vi "CH_LM Config Position Stability Cycle Duration.vi"(0 "Meter Index":i32, 2 "Cycle Time (00:01:00)":T1={"Hours"=0, "Minutes"=1, "Seconds"=0}, 5 "error in (no error)":errorcluster, 7 "Timeout / ms (3000)":i32=3000, 8 "Action (query)":bool, 9 "Lock Timeout / ms (1000)":i32=1000) -> (11 "Lock timed out":bool, 14 "Meter Index":i32, 16 "Cycle Time":T1={"Hours"=0, "Minutes"=1, "Seconds"=0}, 19 "error out":errorcluster)   [LabVIEW 2012, in "CH_LM.lvlib"]
doc: "This command will set/query the position stability cycle time, which takes effect at the end of the current position stability cycle.\n\n<B>Attention:</B> This command will apply only when a quadrant thermopile probe is attached in one of the position stability display modes."
uses:
  CH_LM.lvlib
  CH_LM Time.ctl
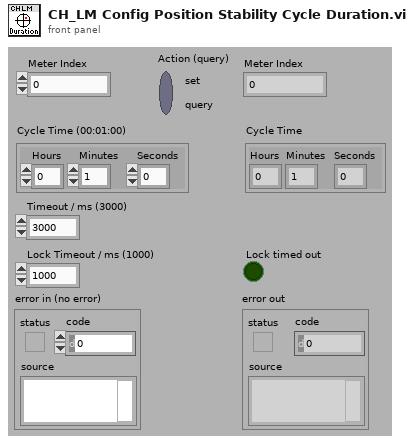
[diagram p1: front panel]
types:
  T1 = typedef "CH_LM.lvlib/CH_LM Time.ctl" = cluster{"Hours":i32, "Minutes":i32, "Seconds":i32}
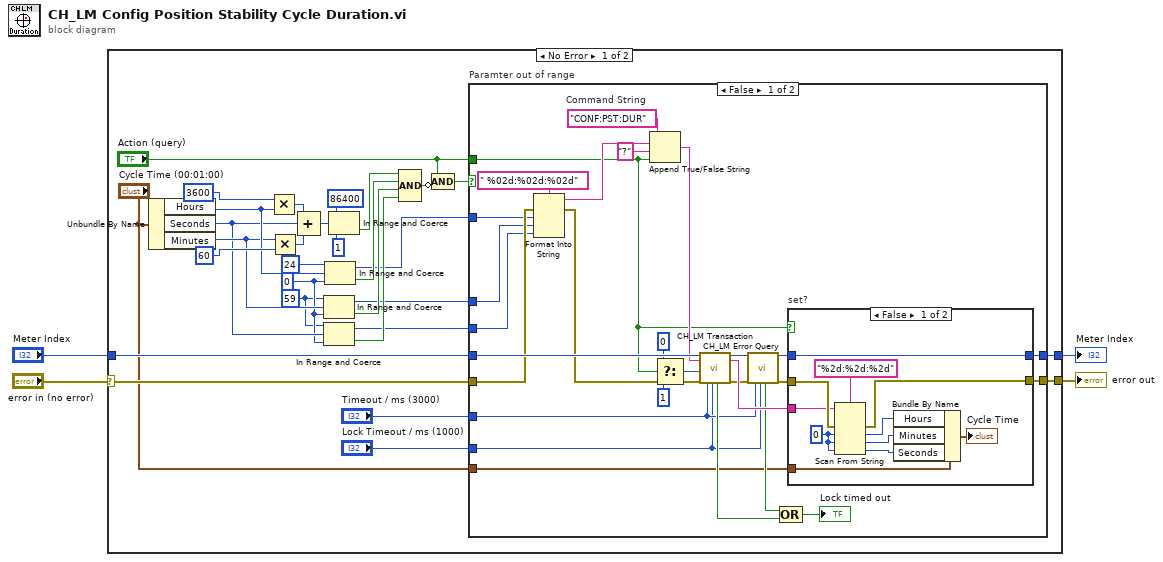
[diagram p0: block diagram]
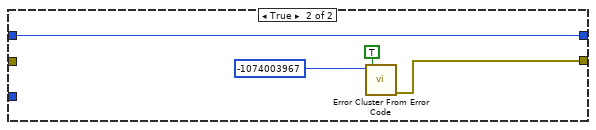
[diagram p3: hidden frame]
diagram:
  n1 = case shown="No Error" "error in (no error)" {
    selector: "error in (no error)" -> [w34 w81]
    tunnel: [w32 w81] -> w4
    tunnel: "Meter Index" -> [w33 w80]
    tunnel: [w31 w80] -> w1
    frame No Error {
      w13 = 59 ("upper limit")
      w14 = 0 ("lower limit")
      n2 = Unbundle By Name("Cycle Time (00:01:00)") -> ("Hours"=w17:i32, "Seconds"=w15:i32, "Minutes"=w16:i32)
      n3 = Multiply(x=3600, y=w17) -> (x*y=w23:i32)
      n4 = Multiply(x=w16, y=60) -> (x*y=w22:i32)
      n5 = Compound Arithmetic op=ADD(w23, w15, w22) -> (w21:i32)
      n6 = In Range and Coerce(upper limit=w13, x=w16, lower limit=w14) -> (coerced(x)=w6:i32, In Range?=w9:bool)
      n7 = In Range and Coerce(upper limit=w13, x=w15, lower limit=w14) -> (coerced(x)=w5:i32, In Range?=w8:bool)
      n8 = In Range and Coerce(upper limit=24, x=w17, lower limit=w14) -> (coerced(x)=w7:i32, In Range?=w10:bool)
      n9 = In Range and Coerce(upper limit=86400, x=w21, lower limit=1) -> (In Range?=w11:bool)  [unwired: 1 out]
      n10 = Compound Arithmetic op=AND(w11, w10, w9, w8) -> (w12:bool)
      n11 = Compound Arithmetic op=AND("Action (query)", invert w12) -> (w26:bool)
      n12 = case "Paramter out of range" shown="False" w26 {
        tunnel: w34 -> [w50 _]
        tunnel: w33 -> [w62 w79]
        tunnel: [w59 w77] -> w32
        tunnel: [w56 w79] -> w31
        tunnel: "Timeout / ms (3000)" -> [w42 _]
        tunnel: "Lock Timeout / ms (1000)" -> [w41 _]
        tunnel: w7 -> [w47 _]
        tunnel: "Action (query)" -> [w39 _]
        tunnel: "Cycle Time (00:01:00)" -> [w43 _]
        tunnel: w6 -> [w45 _]
        tunnel: w5 -> [w44 _]
        frame False {
          w61 = "CONF:PST:DUR"  # Command String
          n13 = Format Into String(format string=" %02d:%02d:%02d", error in=w50, w47, w45, w44) -> (resulting string=w48:string, error out=w37:errorcluster)  [unwired: 1 in]
          n14 = Append True/False String(1:w39, 2:"?" ("true string"), 3:w48, 4:w61) -> (0:w49:string)
          n15 = Select(t=0, s=w39, f=1 ("NofStrings (-1:all)")) -> (s? t:f=w40:i32)
          n16 = call "CH_LM Transaction.vi"("Meter Index"=w62, "Command String"=w49, "NofStrings (-1:all)"=w40, "error in (no error)"=w37, "Timeout / ms (3000)"=w42, "Lock Timeout / ms (1000)"=w41) -> ("Lock timed out"=w52:bool, "Meter Index"=w36:i32, "Response"=w60:string, "error out"=w35:errorcluster)  [unwired: 10 out]
          n17 = call "CH_LM Error Query.vi"("Meter Index"=w36, "error in (no error)"=w35, "Timeout / ms (3000)"=w42, "Lock Timeout / ms (1000)"=w41) -> ("Lock timed out"=w53:bool, "Meter Index"=w55:i32, "error out"=w54:errorcluster)  [unwired: 13 out]
          n18 = Compound Arithmetic op=OR(w53, w52) -> (→"Lock timed out":bool)
          n19 = case "set?" shown="False" w39 {
            tunnel: w60 -> [w70 _]
            tunnel: w54 -> [w73 w75]
            tunnel: [w72 w75] -> w59
            tunnel: w55 -> [w71 w74]
            tunnel: [w71 w74] -> w56
            tunnel: w43 -> [w67 _]
            frame False {
              w69 = 0 ("default value 1")
              n20 = Scan From String(format string="%2d:%2d:%2d", input string=w70, error in=w73, default 1=w69, default 2=w69, default 3=w69) -> (error out=w72:errorcluster, output 1=w66:i32, output 2=w65:i32, output 3=w64:i32)  [unwired: 1 in, 2 out]
              n21 = Bundle By Name(cluster=w67, "Hours"=w66, "Minutes"=w65, "Seconds"=w64) -> (→"Cycle Time":T1)
            }
            frame True {
            }
          }
        }
        frame True {
          n22 = call <vilib>:"Error Cluster From Error Code.vi"("show call chain? (False)"=TRUE, "error code (0)"=-1074003967) -> ("error out"=w77:errorcluster)  [unwired: 1 in, 6 out]
        }
      }
    }
    frame Error {
    }
  }
  "error out" <- w4
  "Meter Index" <- w1
